vi "Read Spell.vi"(8 "error in (no error)":errorcluster, 11 "EnchantedRoom in":refnum<class "EnchantedRoom.lvclass">) -> (0 "error out":errorcluster, 2 "Spell*":refnum<data-value>, 3 "EnchantedRoom out":refnum<class "EnchantedRoom.lvclass">)   [LabVIEW 2016, in "EnchantedRoom.lvclass"]
uses:
  EnchantedRoom.lvclass
  Spell/Spell.lvclass
  EnchantedRoom.lvclass/EnchantedRoom.ctl
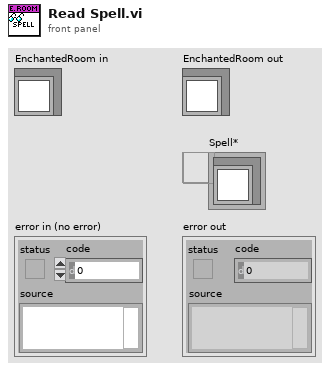
[diagram p1: front panel]
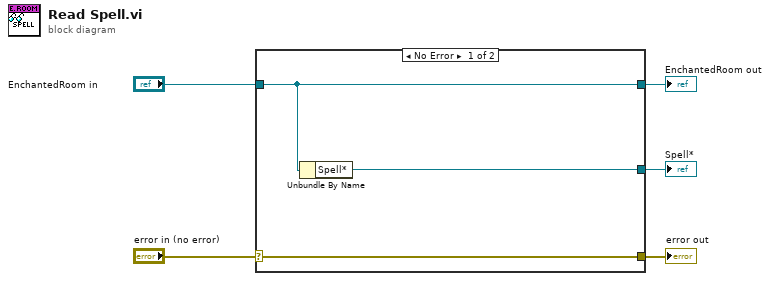
[diagram p0: block diagram]
diagram:
  n1 = case shown="No Error" "error in (no error)" {
    selector: "error in (no error)" -> [w8 w9]
    tunnel: [w8 w9] -> w4
    tunnel: [w7 w10] -> w2
    tunnel: "EnchantedRoom in" -> [w7 w10]
    tunnel: [w6 _] -> w1
    frame No Error {
      n2 = Unbundle By Name(w7) -> ("Spell*"=w6:refnum<data-value>)
    }
    frame Error {
    }
  }
  "error out" <- w4
  "EnchantedRoom out" <- w2
  "Spell*" <- w1
